vi "Parse CLI Inputs GoCD.vi"(10 "Custom Parameters":string[](array[string]), 11 "Working Directory":path) -> (0 "error out":errorcluster, 2 "CLI Inputs":T1, 3 "Library Name":string)   [LabVIEW 2019]
uses:
  CLI-Inputs.ctl
  TargetType.ctl
  <vilib>/Wiresmith Technology/G CLI/CLI Class/CLI.lvclass
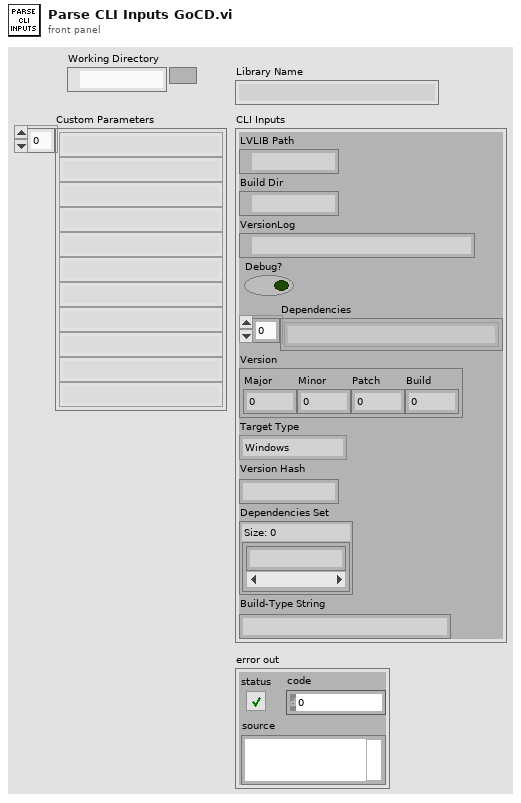
[diagram p1: front panel]
types:
  T1 = typedef "CLI-Inputs.ctl" = cluster{"LVLIB Path":path, "Build Dir":path, "VersionLog":path, "Debug?":bool, "Dependencies":string[], "Version":cluster{"Major":i32, "Minor":i32, "Patch":i32, "Build":i32}, "Target Type":T2, "Version Hash":string, "Dependencies Set":set{string}, "Build Type":string}
  T2 = typedef "TargetType.ctl" = enum16{"Windows", "cRIO-9045"}
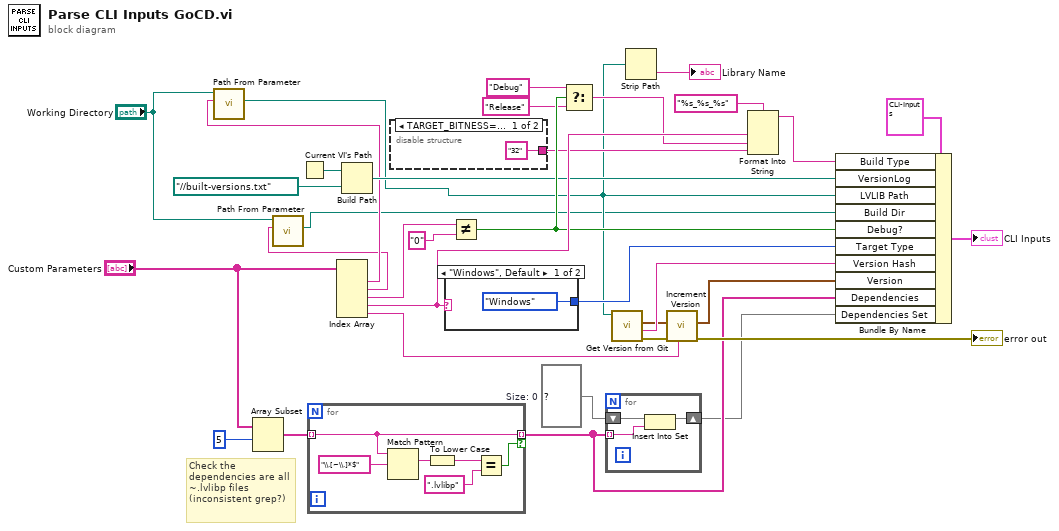
[diagram p0: block diagram]
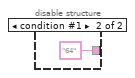
[diagram p2: hidden frame]
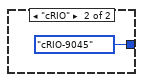
[diagram p3: hidden frame]
diagram:
  w19 = set{string} {}  # Size: 0
  # "Check the dependencies are all ~.lvlibp files (inconsistent grep?)"
  n1 = Array Subset(array="Custom Parameters", index=5) -> (w31:string[])  [unwired: 1 in]
  n2 = Current VI's Path() -> (path=w14:path)
  n3 = for {
    tunnel: w31 -> [w36] mode=indexing
    tunnel: [w36] -> w20 mode=indexing if=w35
    n4 = Match Pattern(string=w36, regular expression="\\.[~\\.]*$") -> (match substring=w39:string)  [unwired: 4 out]
    n5 = To Lower Case(string=w39) -> (all lower case string=w40:string)
    n6 = Equal?(x=w40, y=".lvlibp") -> (x = y?=w35:bool)
  }
  n7 = Index Array(array="Custom Parameters") -> (element #1=w5:string, element #2=w3:string, element #3=w17:string, element #4=w34:string, element #5=w16:string)  [unwired: 5 in]
  n8 = call <vilib>:"Path From Parameter.vi"("Path Parameter"=w5, "Working Directory"="Working Directory") -> ("Full Path"=w4:path)  [unwired: 9 in]
  n9 = call <vilib>:"Path From Parameter.vi"("Path Parameter"=w3, "Working Directory"="Working Directory") -> ("Full Path"=w1:path)  [unwired: 9 in]
  n10 = Build Path(base path=w14, name or relative path=path "../../built-versions.txt" ("VersionLog")) -> (appended path=w12:path)
  n11 = disable-structure shown="TARGET_BITNESS==32, Default" {
    disable-tunnel: ["32" "64"] -> w6
    frame condition #0 (active) {
    }
    frame condition #1 {
    }
  }
  n12 = case shown="\"Windows\", Default" w34 {
    tunnel: [TargetType."Windows" ("Target Type") TargetType."cRIO-9045" ("Target Type")] -> w33
    frame "Windows", Default {
    }
    frame "cRIO" {
    }
  }
  n13 = Not Equal?(x=w17, y="0") -> (x != y?=w32:bool)
  n14 = Select(t="Debug", s=w32, f="Release") -> (s? t:f=w7:string)
  n15 = for {
    tunnel: w20 -> [w46] mode=indexing
    shift-right: [w45] -> w18
    shift-left: w19 -> [w47]
    n16 = Insert Into Set(10:w46, 11:w47) -> (3:w45:set{string})  [unwired: 1 out]
  }
  n17 = call "Get Version from Git.vi"("lvlib path"=w4) -> ("error out"=w23:errorcluster, "Commit Hash"=w25:string, "Version"=w24:cluster{i32, i32, i32, i32})  [unwired: 8 in]
  n18 = Strip Path(path=w4) -> (name=→"Library Name":string)  [unwired: 1 out]
  n19 = call "Increment Version.vi"("Revision Type String"=w16, "error in (no error)"=w23, "Previous Version"=w24) -> ("error out"=→"error out":errorcluster, "New Version"=w21:cluster{i32, i32, i32, i32})  [unwired: 7 in]
  n20 = Format Into String(format string="%s_%s_%s", w34, w7, w6) -> (resulting string=w11:string)  [unwired: 2 in, 1 out]
  n21 = Bundle By Name(cluster=T1 {"LVLIB Path"=path "", "Build Dir"=path "", "VersionLog"=path "", "Debug?"=FALSE, "Dependencies"=[], "Version"={"Major"=0, "Minor"=0, "Patch"=0, "Build"=0}, "Target Type"=enum."Windows", "Version Hash"="", "Dependencies Set"={}, "Build Type"=""} ("Cluster"), "Build Type"=w11, "VersionLog"=w12, "LVLIB Path"=w4, "Build Dir"=w1, "Debug?"=w32, "Target Type"=w33, "Version Hash"=w25, "Version"=w21, "Dependencies"=w20, "Dependencies Set"=w18) -> (→"CLI Inputs":T1)
